vi "UpdateCVT(SetTrigger).vi"(8 "error in (no error)":errorcluster, 11 "TektronixDPO in":refnum<class "TektronixDPO.lvclass">) -> (0 "error out":errorcluster, 3 "TektronixDPO out":refnum<class "TektronixDPO.lvclass">)   [LabVIEW 2013, in "TektronixDPO.lvclass"]
uses:
  TektronixDPO.lvclass
  TektronixDPO.lvclass/TektronixDPO.ctl
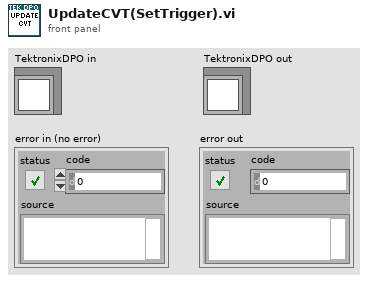
[diagram p1: front panel]
types:
  T1 = typedef "TriggerCluster.ctl" = cluster{"Mode":T2, "Source":T3, "Coupling":T4, "Slope":T5, "Low Level":dbl}
  T2 = typedef "Choice73.ctl" = enum16{"Immediate", "Analog Edge"}
  T3 = typedef "Choice74.ctl" = enum16{"Channel 1", "Channel 2", "Channel 3", "Channel 4", "AC Line", "Aux", "Digital Channel 0", "Digital Channel 1", "Digital Channel 2", "Digital Channel 3", "Digital Channel 4", "Digital Channel 5", "Digital Channel 6", "Digital Channel 7", "Digital Channel 8", "Digital Channel 9", "Digital Channel 10", "Digital Channel 11", "Digital Channel 12", "Digital Channel 13", "Digital Channel 14", "Digital Channel 15", "RF"}
  T4 = typedef "Choice75.ctl" = enum16{"DC", "HF Reject", "LF Reject", "Noise Reject", "AC"}
  T5 = typedef "Choice76.ctl" = enum16{"Rising", "Falling"}
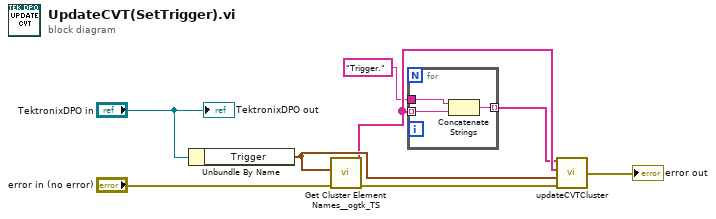
[diagram p0: block diagram]
diagram:
  n1 = Unbundle By Name("TektronixDPO in") -> ("Trigger"=w8:T1)
  n2 = call "Get Cluster Element Names__ogtk_TS.vi"("error in (no error)"="error in (no error)", "Variant"=w8) -> ("error out"=w7:errorcluster, "Names (Array)"=w4:string[])  [unwired: 8 in]
  n3 = for {
    tunnel: w4 -> [w11] mode=indexing
    tunnel: "Trigger." -> [w10]
    tunnel: [w9] -> w2 mode=indexing
    n4 = Concatenate Strings(w10, w11) -> (w9:string)
  }
  n5 = call "updateCVTCluster.vi"("error in"=w7, "variant (destination) out"=w8, "Cluster Names"=w4, "CVT Names"=w2) -> ("error out"=→"error out":errorcluster)
  "TektronixDPO out" <- "TektronixDPO in"
